vi "To CSV File.vi"(8 "error in":errorcluster, 9 "Path":path, 10 "engine configuration":refnum<class "engine configuration.lvclass">, 11 "SystemLink editor node in":refnum<class "SystemLink editor node.lvclass">) -> (0 "error out":errorcluster, 3 "SystemLink editor node out":refnum<class "SystemLink editor node.lvclass">)   [LabVIEW 2015, in "SystemLink editor node.lvclass"]
uses:
  SystemLink editor node.lvclass
  <vilib>/NI/Module Execution Interface/Engine Configuration/engine configuration.lvclass
  module/configuration/SystemLink configuration.lvclass
  <vilib>/NI/Configuration Framework/serializable configuration/NISE_CEF_serializable configuration.lvclass/NISE_CEF_serializable configuration.ctl
  module/configuration/SystemLink configuration.lvclass/SystemLink configuration.ctl
  <vilib>/NI/Tag Bus/tag/tag descriptor.lvclass/tag descriptor.ctl
  <vilib>/Utility/LVClass/Get LV Class Name.vi
  <vilib>/NI/Configuration Framework/error generator/NISE_error generator.vi
  <vilib>/NI/Tag Bus Module Framework/channel/TBM channel.lvclass
  <vilib>/NI/Configuration Framework/serializable configuration/NISE_CEF_serializable configuration.lvclass
  <vilib>/NI/Tag Bus/tag/tag descriptor.lvclass
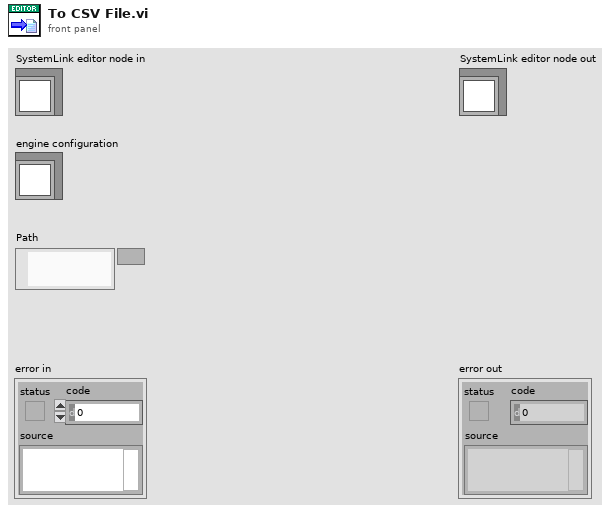
[diagram p1: front panel]
types:
  T1 = typedef "SystemLink configuration.lvclass/Line.ctl" = cluster{"channel":refnum<class "TBM channel.lvclass">}
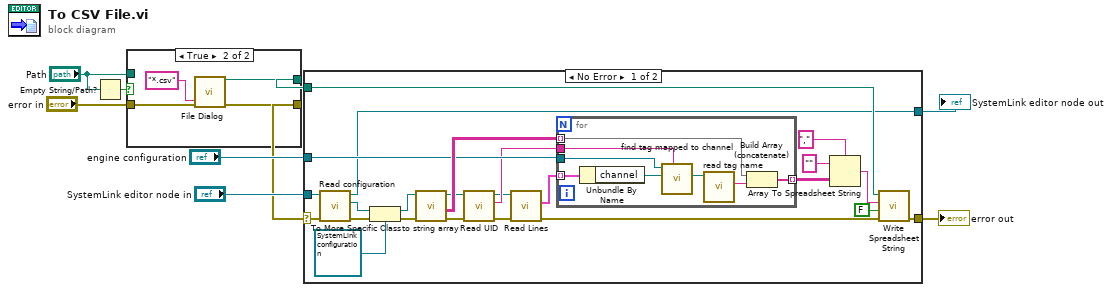
[diagram p0: block diagram]
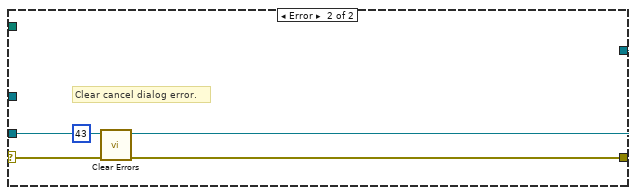
[diagram p2: hidden frame]
diagram:
  n1 = Empty String/Path?(string/path="Path") -> (empty?=w9:bool)
  n2 = case shown="True" w9 {
    tunnel: "error in" -> [w10 w14]
    tunnel: [w10 w13] -> w2
    tunnel: [w11 w12] -> w3
    tunnel: "Path" -> [w11 _]
    frame False {
    }
    frame True {
      n3 = call "File Dialog"("error in"=w14, "pattern (all files)"="*.csv") -> ("selected path"=w12:path, "error out"=w13:errorcluster)  [unwired: 10 in, 2 out]
    }
  }
  n4 = case shown="No Error" w2 {
    selector: w2 -> [w26 w50]
    tunnel: [w37 w49] -> w1
    tunnel: [w25 w51] -> w6
    tunnel: "SystemLink editor node in" -> [w27 w51]
    tunnel: w3 -> [w33 _]
    tunnel: "engine configuration" -> [w30 _]
    frame No Error {
      n5 = call-dynamic "Read configuration.vi"("error in"=w26, "SystemLin Tag Module editor node in"=w27) -> ("error out"=w24:errorcluster, "configuration"=w23:refnum<class "NISE_CEF_serializable configuration.lvclass">, "SystemLin Tag Module editor node out"=w25:refnum<class "SystemLink editor node.lvclass">)  [unwired: 7 in]
      n6 = To More Specific Class(target class=refnum<class "SystemLink configuration.lvclass"> refnum ("SystemLin Tag Module configuration"), reference=w23, error in=w24) -> (specific class reference=w39:refnum<class "SystemLink configuration.lvclass">, error out=w38:errorcluster)
      n7 = call-dynamic "to string array.vi"("error in (no error)"=w38, "module configuration in"=w39) -> ("error out"=w18:errorcluster, "Array"=w32:string[][], "module configuration out"=w19:refnum<class "SystemLink configuration.lvclass">)  [unwired: 6 in, 1 out]
      n8 = call <vilib>:"Read UID.vi"("error in"=w18, "configuration in"=w19) -> ("error out"=w17:errorcluster, "instance id"=w29:string, "configuration out"=w20:refnum<class "SystemLink configuration.lvclass">)  [unwired: 7 in]
      n9 = call "Read Lines.vi"("error in (no error)"=w17, "SystemLin Tag Module configuration in"=w20) -> ("error out"=w16:errorcluster, "Lines"=w21:T1[])  [unwired: 7 in, 1 out]
      n10 = for {
        tunnel: w32 -> [w43] mode=indexing
        tunnel: [w41] -> w31 mode=indexing
        tunnel: w21 -> [w47] mode=indexing
        tunnel: w30 -> [w45]
        tunnel: w29 -> [w40]
        n11 = Unbundle By Name(w47) -> ("channel"=w46:refnum<class "TBM channel.lvclass">)
        n12 = call <vilib>:"find tag mapped to channel.vi"("owner"=w40, "channel"=w46, "engine configuration in"=w45) -> ("tag"=w44:refnum<class "tag descriptor.lvclass">)  [unwired: 6 in, 2 out]
        n13 = call <vilib>:"read tag name.vi"("system tag in"=w44) -> ("name"=w42:string)  [unwired: 8 in, 2 out]
        n14 = Build Array (concatenate)(w43, w42) -> (w41:string[])
      }
      n15 = Array To Spreadsheet String(delimiter (Tab)=",", array=w31, 3:"" ("format string")) -> (spreadsheet string=w36:string)
      n16 = call <vilib>:"Write Spreadsheet String.vi"("error in"=w16, "append to file? (new file:F)"=FALSE, "spreadsheet string"=w36, "file path (dialog if empty)"=w33) -> ("error out"=w37:errorcluster)  [unwired: 6 in, 1 out]
    }
    frame Error {
      # "Clear cancel dialog error."
      n17 = call <vilib>:"Clear Errors.vi"("error in (no error)"=w50, "specific error code to clear (0: all)"=43) -> ("error out"=w49:errorcluster)  [unwired: 4 in, 1 out]
    }
  }
  "error out" <- w1
  "SystemLink editor node out" <- w6
